vi "Get MCP Gain Range.vi"(10 "iHigh":i32, 11 "iLow":i32) -> (1 "function return":u32, 2 "iHigh out":i32, 3 "iLow out":i32)   [LabVIEW 2018, in "Copy of Andor SDK.lvlib"]
doc: "EXPNETTYPE unsigned int WINAPI GetMCPGainRange(int * iLow, int * iHigh);"
uses:
  Copy of Andor SDK.lvlib
  <userlib>/Andor SDK/ATMCD32D.dll
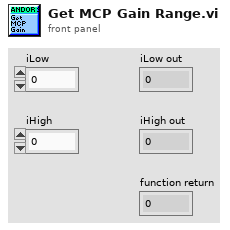
[diagram p1: front panel]
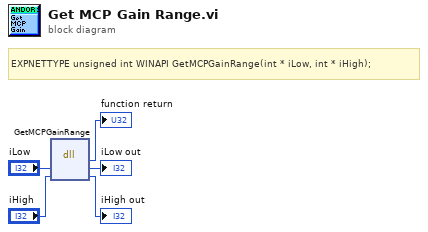
[diagram p0: block diagram]
diagram:
  # "EXPNETTYPE unsigned int WINAPI GetMCPGainRange(int * iLow, int * iHigh);"
  n1 = dll-call lib="C:/Program Files (x86)/National Instruments/LabVIEW 2018/user.lib/Andor SDK/ATMCD32D.*" fn="GetMCPGainRange"("iLow"="iLow", "iHigh"="iHigh") -> (→"function return":u32, "iLow"=→"iLow out":i32, "iHigh"=→"iHigh out":i32)  [unwired: 3 in, 2 out]
